vi "Search For VI.vi"(8 "Error In":errorcluster, 10 "VI Filename To Search For":string, 11 "DFS Data In":T1) -> (0 "Error Out":errorcluster, 1 "VI's ProjectItem Ref":refnum<vi>, 2 "VI Found?":bool, 3 "DFS Data Out":T1)   [LabVIEW 2022 SP3]
doc: "<add documentation here>"
uses:
  DFS Data (cluster).ctl
  DFS Node (cluster).ctl
  DFS Child Node (cluster).ctl
panel:
  # "Development\nControls or indicators that are useful for development or testing, but which are not outputs of the VI."
  # "Input\nInputs to the VI"
  # "Output\nOutputs of the VI"
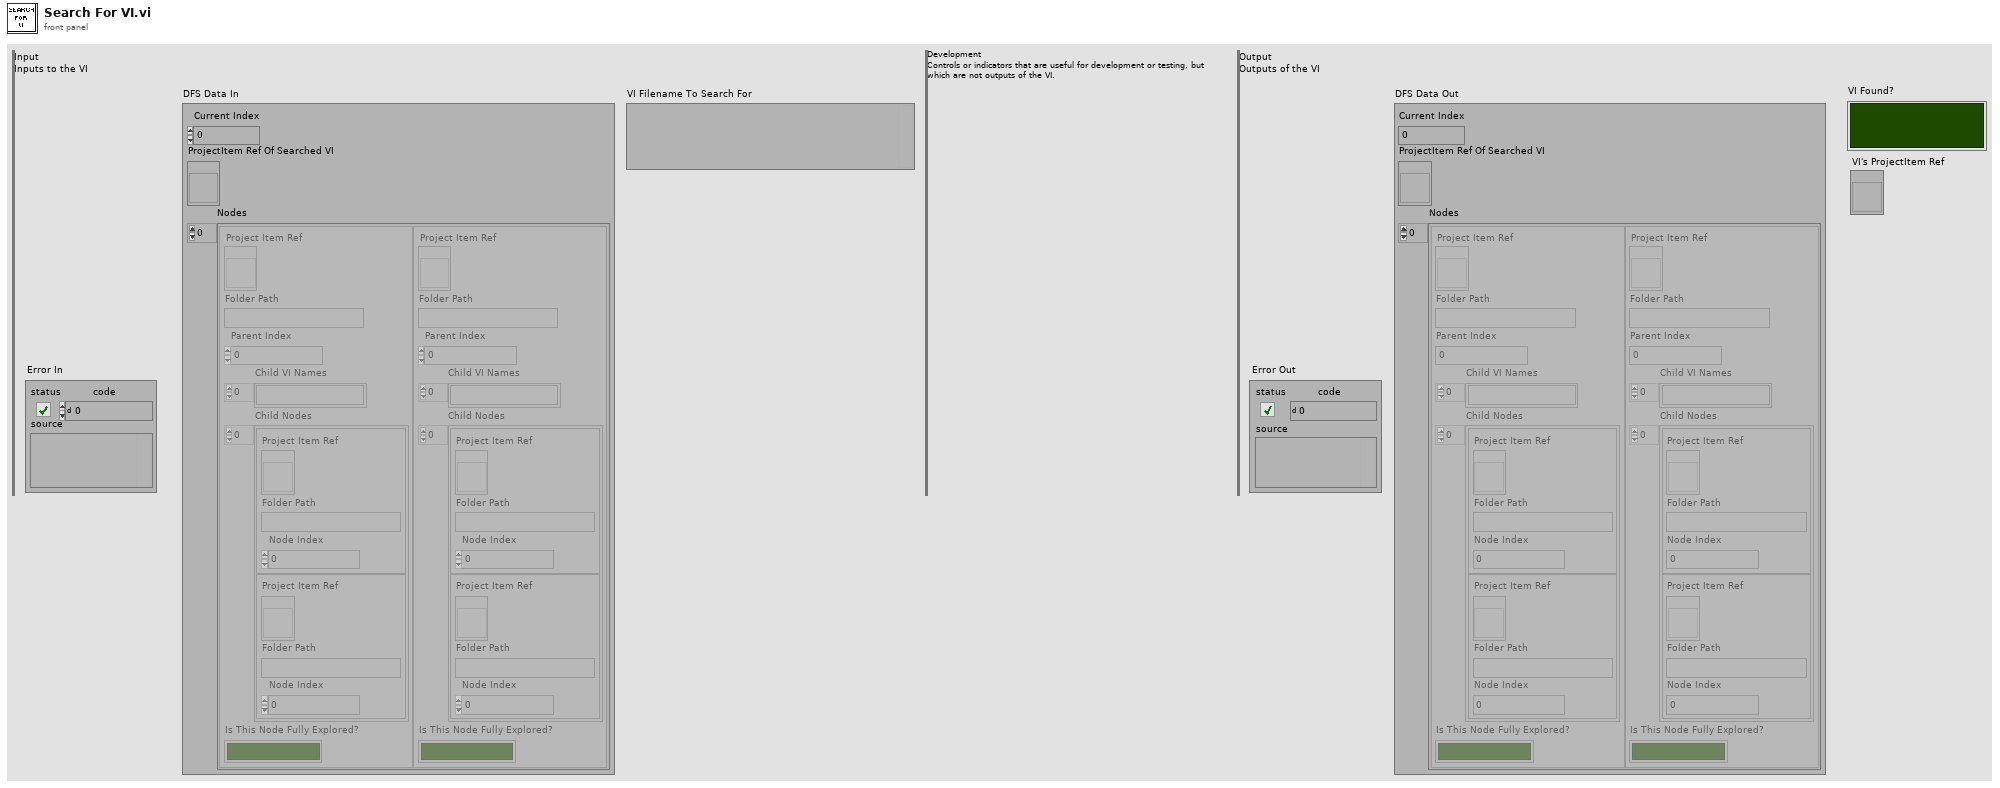
[diagram p1: front panel]
types:
  T1 = typedef "DFS Data (cluster).ctl" = cluster{"Current Index":i32, "ProjectItem Ref Of Searched VI":refnum<vi>, "Nodes":T2[]}
  T2 = typedef "DFS Node (cluster).ctl" = cluster{"Project Item Ref":refnum<vi>, "Folder Path":string, "Parent Index":i32, "Child VI Names":string[], "Child Nodes":T3[], "Is This Node Fully Explored?":bool}
  T3 = typedef "DFS Child Node (cluster).ctl" = cluster{"Project Item Ref":refnum<vi>, "Folder Path":string, "Node Index":i32}
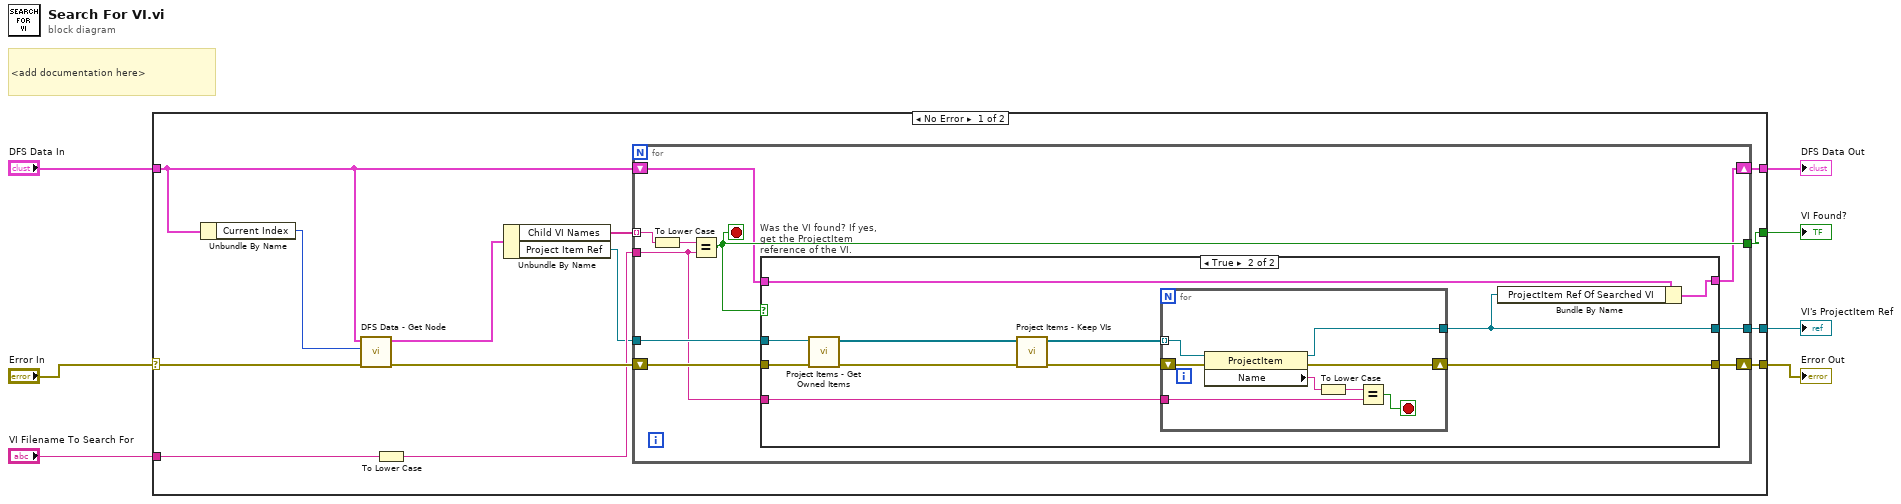
[diagram p0: block diagram]
diagram:
  # "<add documentation here>"
  n1 = case shown="No Error" "Error In" {
    selector: "Error In" -> [w20 w53]
    tunnel: [w12 w53] -> w6
    tunnel: "DFS Data In" -> [w9 w52]
    tunnel: [w8 w52] -> w4
    tunnel: "VI Filename To Search For" -> [w16 _]
    tunnel: [w14 _] -> w2
    tunnel: [w10 _] -> w1
    frame No Error {
      n2 = Unbundle By Name(w9) -> ("Current Index"=w18:i32)
      n3 = call "DFS Data - Get Node.vi"("Error In"=w20, "Node Index"=w18, "DFS Data"=w9) -> ("Error Out"=w19:errorcluster, "DFS Node"=w13:T2)  [unwired: 7 in]
      n4 = To Lower Case(string=w16) -> (all lower case string=w15:string)
      n5 = Unbundle By Name(w13) -> ("Child VI Names"=w17:string[], "Project Item Ref"=w11:refnum<vi>)
      n6 = for {
        shift-right: [w27] -> w12
        shift-left: w19 -> [w28]
        tunnel: w17 -> [w30] mode=indexing
        tunnel: w15 -> [w24]
        tunnel: [w25] -> w14
        tunnel: w11 -> [w26]
        tunnel: [w23] -> w10
        shift-right: [w21] -> w8
        shift-left: w9 -> [w22]
        stop <- w25 stop-if-true
        n7 = To Lower Case(string=w30) -> (all lower case string=w29:string)
        n8 = Equal?(x=w29, y=w24) -> (x = y?=w25:bool)
        n9 = case "Was the VI found? If yes, get the ProjectItem reference of the VI." shown="True" w25 {
          tunnel: w28 -> [w32 w43]
          tunnel: [w32 w38] -> w27
          tunnel: w26 -> [_ w39]
          tunnel: w24 -> [_ w36]
          tunnel: [_ w34] -> w23
          tunnel: w22 -> [w31 w35]
          tunnel: [w31 w33] -> w21
          frame False {
          }
          frame True {
            n10 = call "Project Items - Get Owned Items.vi"("Error In"=w43, "Project Item"=w39) -> ("Error Out"=w42:errorcluster, "Owned Items"=w40:refnum<vi>[])  [unwired: 8 in]
            n11 = call "Project Items - Keep VIs.vi"("Error In"=w42, "Project Items"=w40) -> ("Error Out"=w41:errorcluster, "Project Items (VIs)"=w37:refnum<vi>[])  [unwired: 8 in]
            n12 = for {
              shift-right: [w50] -> w38
              shift-left: w41 -> [w51]
              tunnel: w37 -> [w49] mode=indexing
              tunnel: w36 -> [w47]
              tunnel: [w44] -> w34
              stop <- w45 stop-if-true
              n13 = property class="ProjectItem"(reference=w49, error in=w51) -> (reference out=w44:refnum<vi>, error out=w50:errorcluster, "Name"=w48:string)
              n14 = To Lower Case(string=w48) -> (all lower case string=w46:string)
              n15 = Equal?(x=w46, y=w47) -> (x = y?=w45:bool)
            }
            n16 = Bundle By Name(cluster=w35, "ProjectItem Ref Of Searched VI"=w34) -> (w33:T1)
          }
        }
      }
    }
    frame Error {
    }
  }
  "Error Out" <- w6
  "DFS Data Out" <- w4
  "VI Found?" <- w2
  "VI's ProjectItem Ref" <- w1
